vi "declination_angle.vi"(1 "Orbital period (days)":dbl=365.0, 2 "Earth's Tilt (¡)":dbl=23.4, 3 "Day of Year (day)":dbl) -> (0 "Declination (rad)":dbl)   [LabVIEW 2012]
panel:
  out "Declination (¼)":dbl
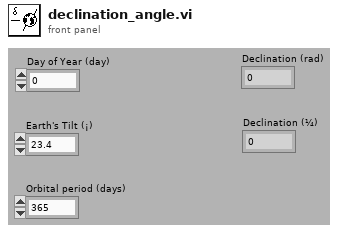
[diagram p1: front panel]
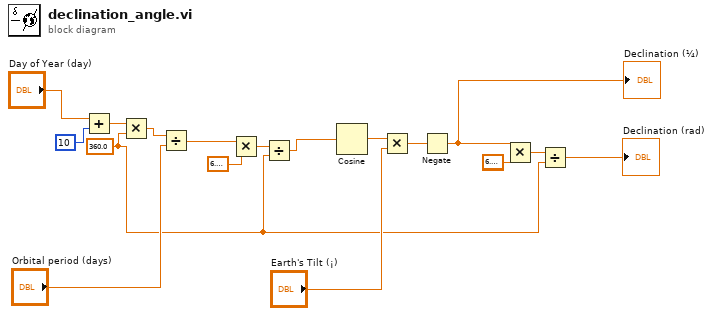
[diagram p0: block diagram]
diagram:
  (unwired) 6.283185307179586
  w4 = 360.0 ("y")
  n1 = Add(x="Day of Year (day)", y=10) -> (x+y=w15:dbl)
  n2 = Multiply(x=w15, y=w4) -> (x*y=w14:dbl)
  n3 = Divide(x=w14, y="Orbital period (days)") -> (x/y=w7:dbl)
  n4 = Multiply(x=w7, y=6.283185307179586) -> (x*y=w5:dbl)
  n5 = Divide(x=w5, y=w4) -> (x/y=w3:dbl)
  n6 = Cosine(x=w3) -> (cos(x)=w12:dbl)
  n7 = Multiply(x=w12, y="Earth's Tilt (¡)") -> (x*y=w10:dbl)
  n8 = Negate(x=w10) -> (-x=w1:dbl)
  "Declination (¼)" <- w1
  n9 = Multiply(x=w1, y=6.283185307179586) -> (x*y=w8:dbl)
  n10 = Divide(x=w8, y=w4) -> (x/y=→"Declination (rad)":dbl)
